vi "Drag & Drop New Multi.vi"(0 "References In":refnum<vi>[](array[refnum]), 1 "Index Panel":i32, 3 "error in":errorcluster) -> (7 "References Out":T1(array[cluster]), 10 "error out":errorcluster)   [LabVIEW 2015]
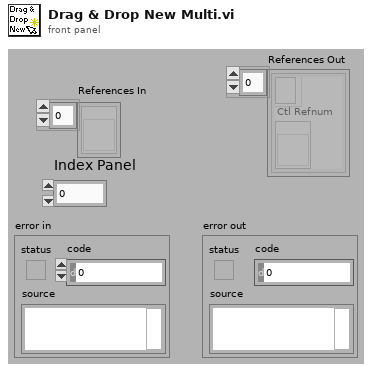
[diagram p1: front panel]
types:
  T1 = cluster{"Event Registration Refnum":refnum<event-registration>, "Ctl Refnum":refnum<vi>}[]
  T2 = cluster{"Event Registration Refnum":refnum<event-registration>, "Ctl Refnum":refnum<vi>}
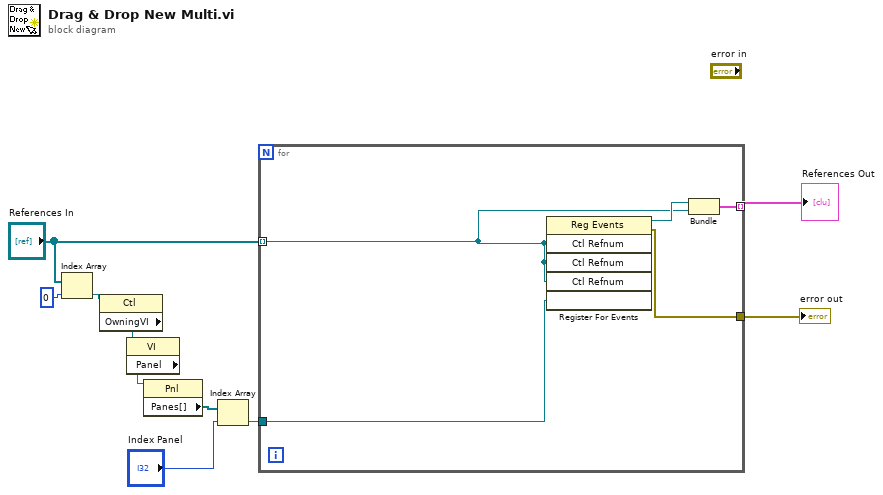
[diagram p0: block diagram]
diagram:
  n1 = Index Array(array="References In", index=0) -> (element=w4:refnum<vi>)
  n2 = property class="Ctl"(reference=w4) -> ("OwningVI"=w5:refnum<vi>)  [unwired: 1 in, 2 out]
  n3 = property class="VI"(reference=w5) -> ("Panel"=w6:refnum<vi>)  [unwired: 1 in, 2 out]
  n4 = property class="Pnl"(reference=w6) -> ("Panes[]"=w2:refnum<vi>[])  [unwired: 1 in, 2 out]
  n5 = Index Array(array=w2, index="Index Panel") -> (element=w1:refnum<vi>)
  n6 = for {
    tunnel: [w15] -> w9
    tunnel: "References In" -> [w12] mode=indexing
    tunnel: [w13] -> w10 mode=indexing
    tunnel: w1 -> [w11]
    n7 = register-events(w12, w12, w12, w11) -> (reference out=w14:refnum<event-registration>, error out=w15:errorcluster)  [unwired: 2 in]
    n8 = Bundle("Event Registration Refnum"=w14, "Ctl Refnum"=w12) -> (w13:T2)  [unwired: 1 out]
  }
  "error out" <- w9
  "References Out" <- w10
